vi "AXIS to POSITION.vi"(9 "Ster pozycyjne":cluster{"X":i16, "Y":i16, "Z":i16}={"X"=100, "Y"=0, "Z"=0} {"Z" scale=0.0..255.0; "Y" scale=0.0..255.0; "X" scale=0.0..255.0}) -> (3 "array of cans":T1[](array[typedef]) {"type" items=["CAN Data", "CAN Remote"]; "identifier" format="%.0x"})   [LabVIEW 2015]
uses:
  RT/CANFrameControl.ctl
panel:
  out "druga ramka manipulator":T1 {"type" items=["CAN Data", "CAN Remote"]; "identifier" format="%.0x"}
  out "Pierwsza ramka manipulator":T1 {"type" items=["CAN Data", "CAN Remote"]; "identifier" format="%.0x"}
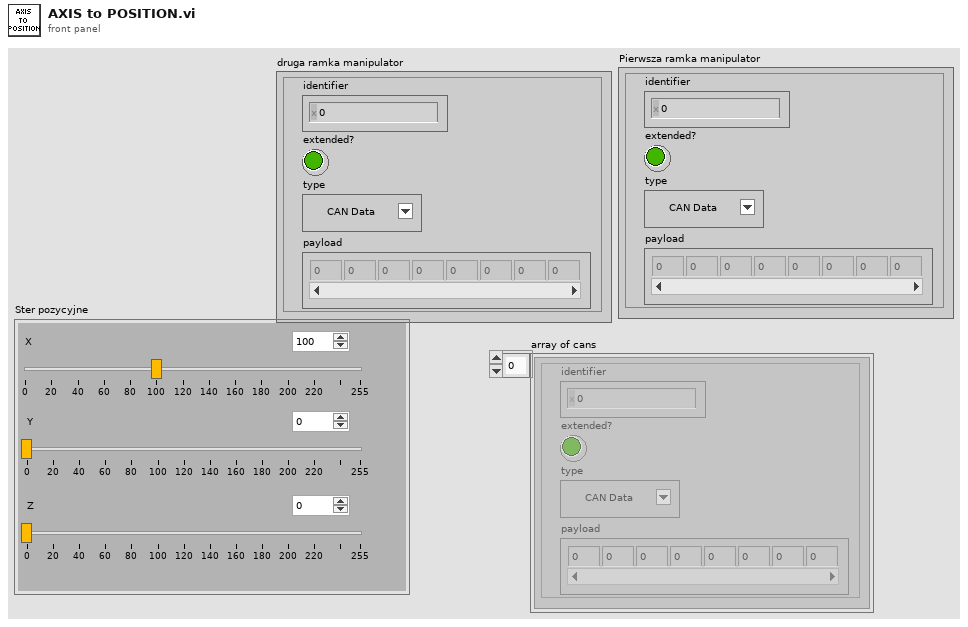
[diagram p1: front panel]
types:
  T1 = typedef "CANFrameControl.ctl" = cluster{"identifier":u32, "extended?":bool, "type":u8, "payload":u8[]}
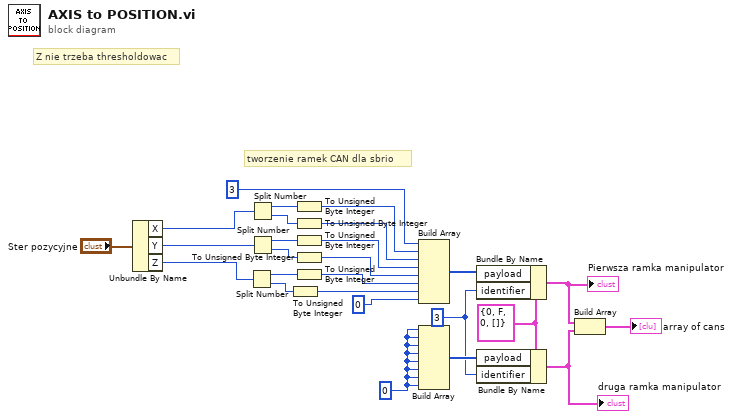
[diagram p0: block diagram]
diagram:
  w6 = u32 3 ("manipulator id")
  w14 = u8 0
  w26 = T1 {"identifier"=0, "extended?"=FALSE, "type"=0, "payload"=[]} ("CAN frame 2")
  # "Z nie trzeba thresholdowac"
  # "tworzenie ramek CAN dla sbrio"
  n1 = Unbundle By Name("Ster pozycyjne") -> ("X"=w3:i16, "Y"=w2:i16, "Z"=w1:i16)
  n2 = Split Number(x=w1) -> (hi(x)=w9:u8, lo(x)=w8:u8)
  n3 = Split Number(x=w3) -> (hi(x)=w13:u8, lo(x)=w12:u8)
  n4 = Split Number(x=w2) -> (hi(x)=w11:u8, lo(x)=w10:u8)
  n5 = To Unsigned Byte Integer(number=w8) -> (unsigned 8bit integer=w16:u8)
  n6 = To Unsigned Byte Integer(number=w13) -> (unsigned 8bit integer=w21:u8)
  n7 = To Unsigned Byte Integer(number=w12) -> (unsigned 8bit integer=w20:u8)
  n8 = To Unsigned Byte Integer(number=w11) -> (unsigned 8bit integer=w19:u8)
  n9 = To Unsigned Byte Integer(number=w10) -> (unsigned 8bit integer=w18:u8)
  n10 = To Unsigned Byte Integer(number=w9) -> (unsigned 8bit integer=w17:u8)
  n11 = Build Array(u8 3 ("zerowy bajt"), w21, w20, w19, w18, w17, w16, u8 0) -> (w15:u8[])
  n12 = Build Array(w14, w14, w14, w14, w14, w14, w14, w14) -> (w25:u8[])
  n13 = Bundle By Name(cluster=w26, "payload"=w15, "identifier"=w6) -> (w23:T1)
  "Pierwsza ramka manipulator" <- w23
  n14 = Bundle By Name(cluster=w26, "payload"=w25, "identifier"=w6) -> (w22:T1)
  "druga ramka manipulator" <- w22
  n15 = Build Array(w23, w22) -> (→"array of cans":T1[])
